vi "Close Motive and PacketClient.vi"(8 "Error In":errorcluster) -> (0 "Error Out":errorcluster)   [LabVIEW 2017]
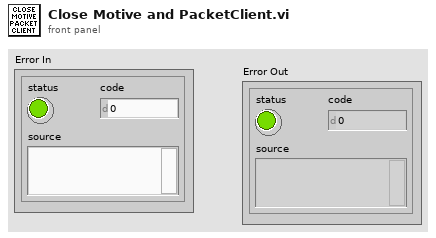
[diagram p1: front panel]
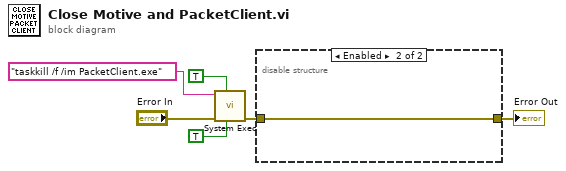
[diagram p0: block diagram]
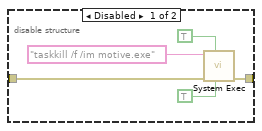
[diagram p2: hidden frame]
diagram:
  n1 = call <vilib>:"System Exec.vi"("run minimized? (F)"=TRUE, "wait until completion? (T)"=TRUE, "error in (no error)"="Error In", "command line"="taskkill /f /im PacketClient.exe" ("String")) -> ("error out"=w3:errorcluster)  [unwired: 4 in, 3 out]
  n2 = disable-structure shown="Enabled" {
    disable-tunnel: w3 -> [w8 w12]
    disable-tunnel: [w7 w12] -> w1
    frame Disabled {
      n3 = call <vilib>:"System Exec.vi"("run minimized? (F)"=TRUE, "wait until completion? (T)"=TRUE, "error in (no error)"=w8, "command line"="taskkill /f /im motive.exe" ("String")) -> ("error out"=w7:errorcluster)  [unwired: 4 in, 3 out]
    }
    frame Enabled {
    }
  }
  "Error Out" <- w1
